vi "UserInterface_API_Init.vi"(8 "error in (no error)":errorcluster, 11 "DataIn":T1) -> (0 "error out":errorcluster)   [LabVIEW 2020]
uses:
  #typedef_UserInterface_Data.ctl
  Cmd_enum.ctl
  #typedef_Parameters_cluster.ctl
  BaudRate_enum.ctl
  Controller/#typedef_ControllerQueue_States.ctl
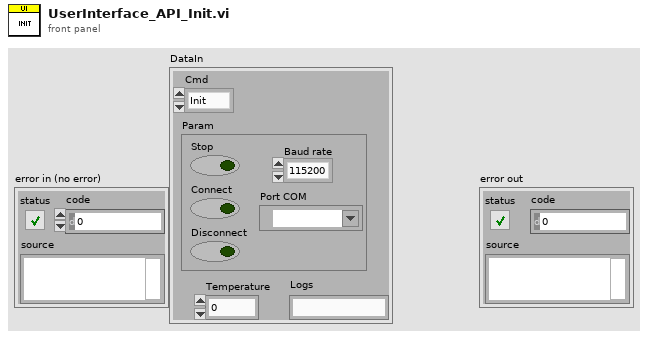
[diagram p1: front panel]
types:
  T1 = typedef "#typedef_UserInterface_Data.ctl" = cluster{"Cmd":T2, "Param":T3, "Temperature":dbl, "Logs":string}
  T2 = typedef "Cmd_enum.ctl" = enum16{"Init", "PrintChart", "Connect", "Disconnect", "ReadData", "Exit"}
  T3 = typedef "#typedef_Parameters_cluster.ctl" = cluster{"Stop":bool, "Connect":bool, "Disconnect":bool, "Port COM":refnum<visa-resource-name>, "Baud rate":T4}
  T4 = typedef "BaudRate_enum.ctl" = enum16{"115200", "9600"}
  T5 = typedef "#typedef_ControllerQueue_States.ctl" = enum16{"Obtain", "GetRef", "Enqueue", "EnqueueAtOpp", "GetStatus", "Flush", "Release"}
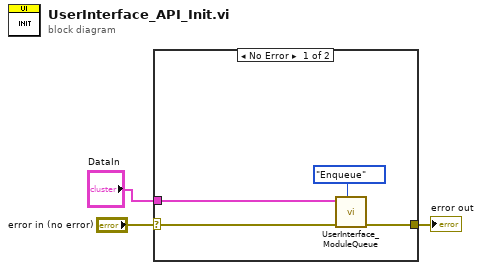
[diagram p0: block diagram]
diagram:
  n1 = case shown="No Error" "error in (no error)" {
    selector: "error in (no error)" -> [w6 w8]
    tunnel: [w7 w8] -> w2
    tunnel: "DataIn" -> [w4 _]
    frame No Error {
      n2 = call "UserInterface_ModuleQueue.vi"(7:#typedef_ControllerQueue_States."Enqueue", "error in (no error)"=w6, "DataIn"=w4) -> ("error out"=w7:errorcluster)  [unwired: 6 in, 2 out]
    }
    frame Error {
    }
  }
  "error out" <- w2
